vi "multifunc_scmos_frame_acquisition.vi"() -> ()   [LabVIEW 2015]
uses:
  <vilib>/Utility/miscctls.llb/LVRectTypeDef.ctl
panel:
  out "Start Trigger Mode":string
  in  "Stop Button":bool
  out "error out":errorcluster
  out "Plot Area Bounds":T1
  out "Image":u16[][](graph)
  in  "Exposure":dbl min=0.0010036691729323308 max=10.000004210526315 step=1e-08
  in  "Scan Mode":dbl min=1.0 max=2.0 step=1.0
  in  "Binning":u16(ring) items=["1x1"=1, "2x2"=2, "4x4"=4]
  out "Exposure":dbl
  out "Scan Mode":dbl
  out "S Vert Width":i32
  out "S Horiz Width":i32
  out "S Vert Offset":i32
  out "S Horiz Offset":i32
  in  "Vertical Width":i32 min=4 max=2048 step=4
  in  "Vertical Offset":i32 min=0 max=0 step=4
  in  "Horizontal Width":i32 min=4 max=2048 step=4
  in  "Horizontal Offset":i32 min=0 max=0 step=4
  in  "Frames":dbl
  out "Timeseries Save Path":path
  out "Snapshot Save Path":path
  out "Timeseries Base Filename":string
  out "Snapshot Base Filename":string
  in  "Timeseries Base Filename":string
  in  "Timeseries Save Path":path
  in  "Snapshot Base Filename":string
  in  "Save Snapshots":bool caption="Save Snapshot"
  in  "Snapshot Save Path":path
  in  "Start Trigger Mode":u32(ring)=1 items=["Internal"=1, "External Edge"=2, "External Level"=4, "Software"=32, "Fast Repetition"=64, "TDI"=128, "Trigger Start"=512, "Sync Readout"=1024]
  out "Model":string
  out "Camera ID":string
  out "Firmware":string
  out "DCAM Ver.":string
  out "Library Ver.":string
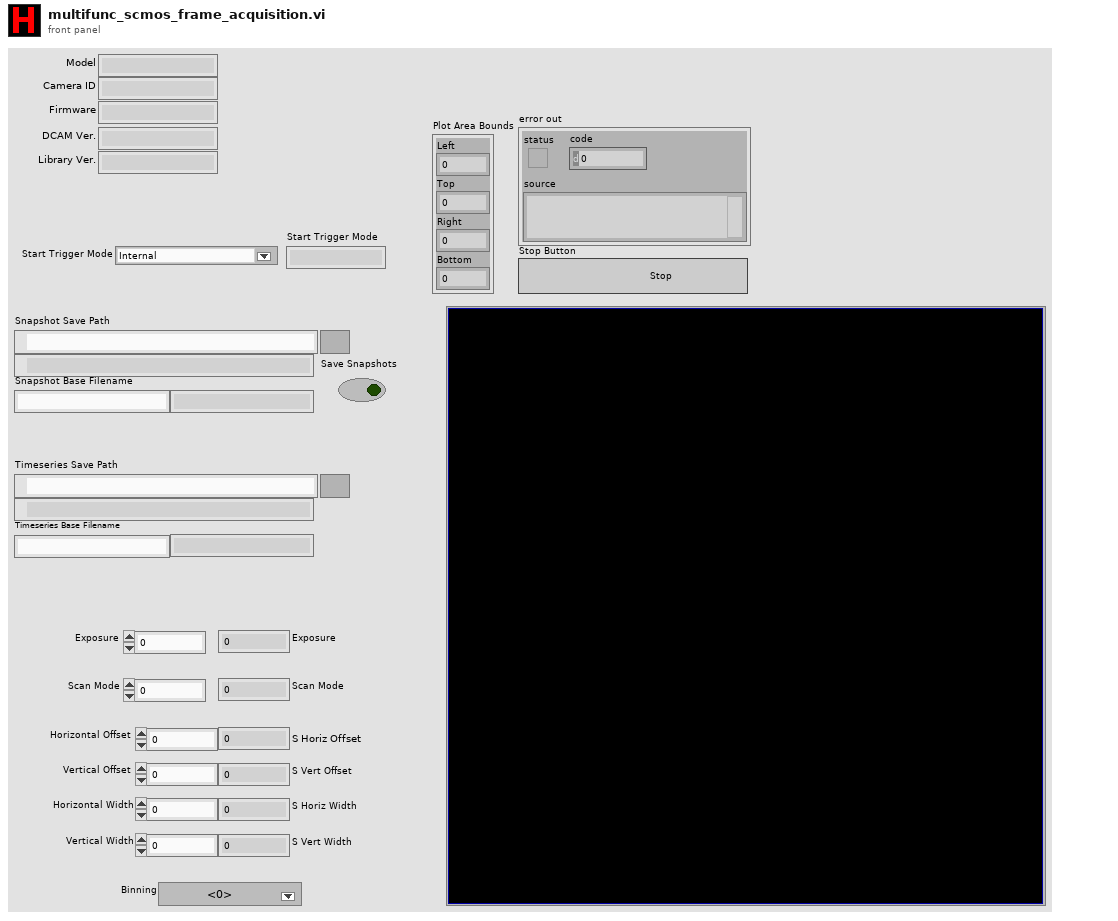
[diagram p1: front panel]
types:
  T1 = typedef "LVRectTypeDef.ctl" = cluster{"Left":i16, "Top":i16, "Right":i16, "Bottom":i16}
  T2 = cluster{"Capture Library":string, "DCAM-API":string}
  T3 = cluster{"Mode":u32, "Polarity":u16, "Times":u32, "Delay":dbl}
  T4 = cluster{"Mode":u32, "Polarity":u32, "Period":dbl, "Delay":dbl}
  T5 = cluster{"Model":string, "Camera ID":string, "Firmware":string}
  T6 = cluster{"Value":i32, "Minimum":i32, "Maximum":i32, "Increment":i32}
  T7 = cluster{"height":u32, "width":u32, "datatype":u32}
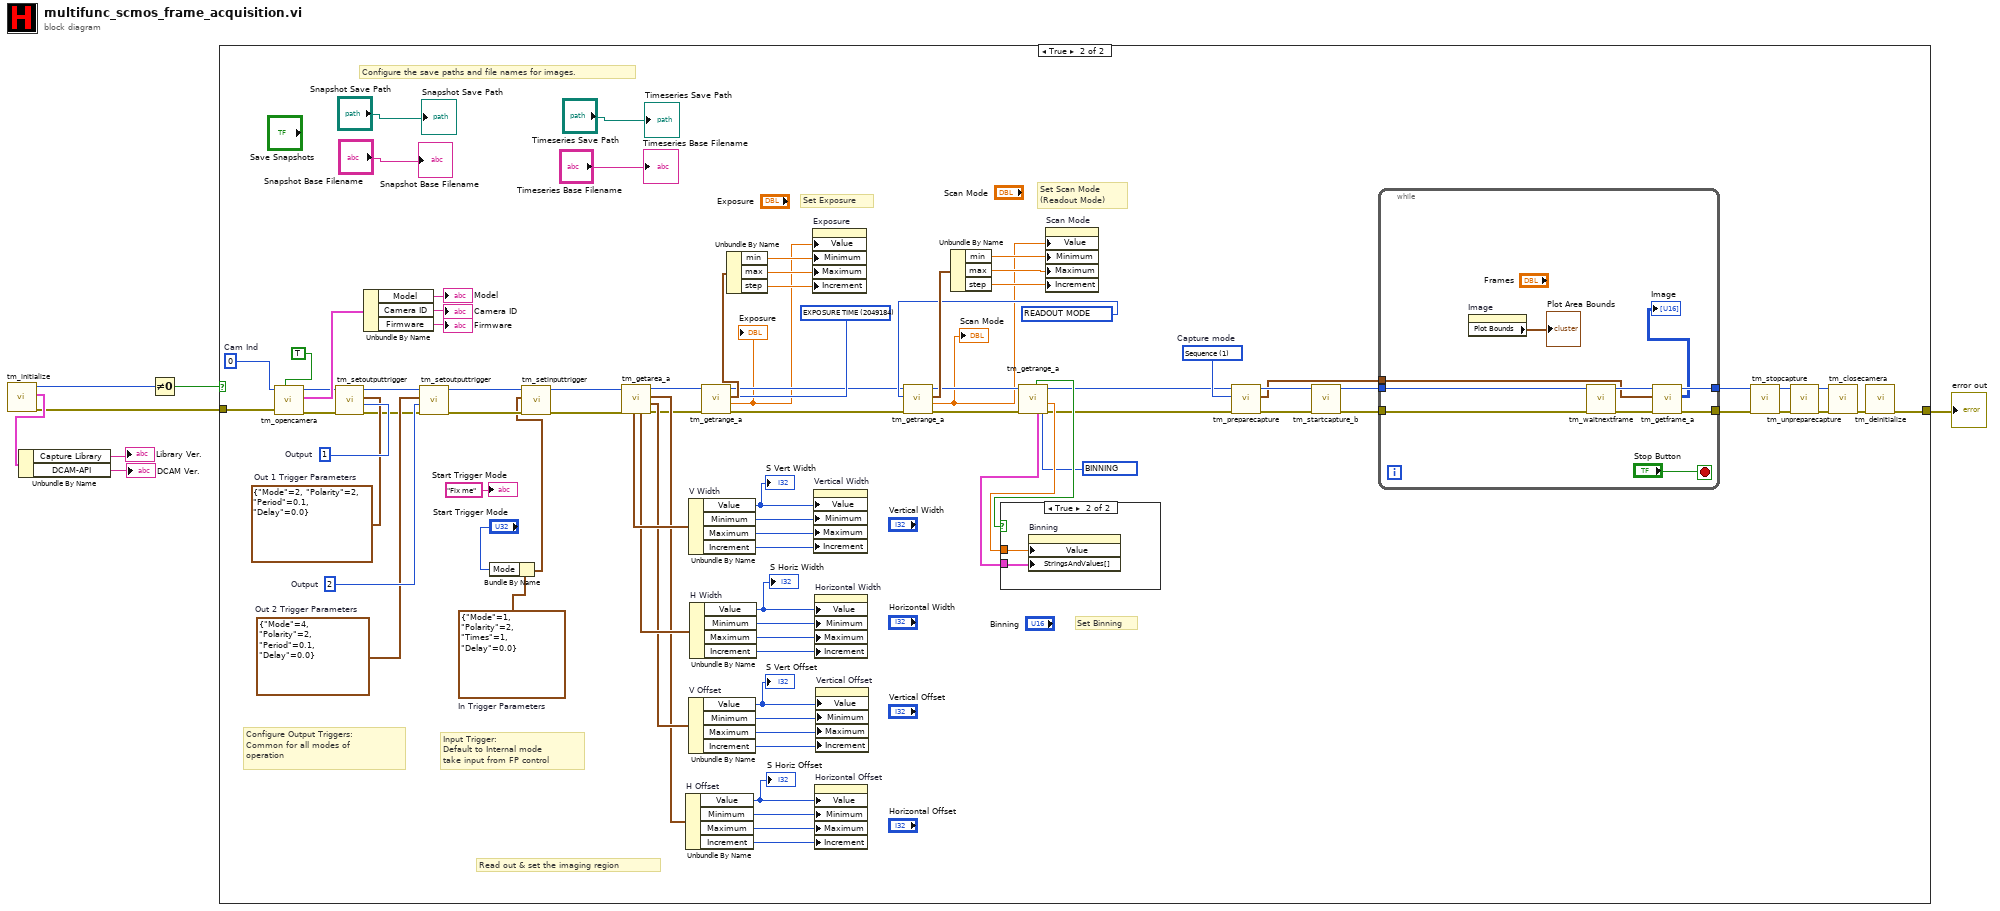
[diagram p0: block diagram]
diagram:
  n1 = call <userlib>:"tm_initialize.vi"() -> ("error out"=w3:errorcluster, "Version Info"=w4:T2, "Number Of Cameras"=w7:u32)  [unwired: 8 in, 1 out]
  n2 = Unbundle By Name(w4) -> ("Capture Library"=→"Library Ver.":string, "DCAM-API"=→"DCAM Ver.":string)
  n3 = Not Equal To 0?(x=w7) -> (x != 0?=w2:bool)
  n4 = case shown="True" w2 {
    tunnel: w3 -> [w8 w80]
    tunnel: [w8 w32] -> w1
    frame False {
    }
    frame True {
      w15 = 1 items=["Snap", "Sequence"]  # Capture mode
      w42 = u32 2049184 items=["BINNING"=4215968, "BITS PER CHANNEL"=4342976, "ACTIVE VIEW INDEX"=4343136, "CCD MODE"=4212384, "SENSOR MODE"=4212128, "READOUT MODE"=4211872, "EXPOSURE TIME"=2049184, "CONTRAST GAIN"=3163312, "CONTRAST OFFSET"=3163328, "LIGHT MODE"=2114720, "SENSITIVITY"=2114992, "WHITE BALANCE"=3163568, "PHOTON IMAGING MODE"=2115200, "HIGH DYNAMIC RANGE MODE"=3163360, "TRIGGER SOURCE"=1066144, "TRIGGER ACTIVE"=1066160, "TRIGGER MODE"=1066400, "TRIGGER POLARITY"=1066416, "TRIGGER GLOBAL EXPOSURE"=2049680, "FIRST TRIGGER BEHAVIOR"=2049696, "TRIGGER TIMES"=1066448, "OUTPUT TRIGGER POLARITY"=1852592, "OUTPUT TRIGGER DELAY"=1852624, "OUTPUT TRIGGER PERIOD"=1852640, "TEMPERATURE"=2115232, "TEMPERATURE TARGET"=2115264, "SENSOR COOLER FAN"=2115296, "MECHANICAL SHUTTER"=2115488, "BACK FOCUS POSITION"=8422304, "FRAMEBUNDLE MODE"=4346784, "FRAMEBUNDLE NUMBER"=4346800, "LINEBUNDLE HEIGHT"=4212192, "TRIGGER CONNECTOR"=1066432, "IMAGE PIXEL TYPE"=4343296, "OUTPUT TRIGGER KIND"=1852656, "READOUT DIRECTION"=4211904, "CHANNEL SYNC"=1852352] ("Parameter")
      w43 = u32 4211872 items=["BINNING"=4215968, "BITS PER CHANNEL"=4342976, "ACTIVE VIEW INDEX"=4343136, "CCD MODE"=4212384, "SENSOR MODE"=4212128, "READOUT MODE"=4211872, "EXPOSURE TIME"=2049184, "CONTRAST GAIN"=3163312, "CONTRAST OFFSET"=3163328, "LIGHT MODE"=2114720, "SENSITIVITY"=2114992, "WHITE BALANCE"=3163568, "PHOTON IMAGING MODE"=2115200, "HIGH DYNAMIC RANGE MODE"=3163360, "TRIGGER SOURCE"=1066144, "TRIGGER ACTIVE"=1066160, "TRIGGER MODE"=1066400, "TRIGGER POLARITY"=1066416, "TRIGGER GLOBAL EXPOSURE"=2049680, "FIRST TRIGGER BEHAVIOR"=2049696, "TRIGGER TIMES"=1066448, "OUTPUT TRIGGER POLARITY"=1852592, "OUTPUT TRIGGER DELAY"=1852624, "OUTPUT TRIGGER PERIOD"=1852640, "TEMPERATURE"=2115232, "TEMPERATURE TARGET"=2115264, "SENSOR COOLER FAN"=2115296, "MECHANICAL SHUTTER"=2115488, "BACK FOCUS POSITION"=8422304, "FRAMEBUNDLE MODE"=4346784, "FRAMEBUNDLE NUMBER"=4346800, "LINEBUNDLE HEIGHT"=4212192, "TRIGGER CONNECTOR"=1066432, "IMAGE PIXEL TYPE"=4343296, "OUTPUT TRIGGER KIND"=1852656, "READOUT DIRECTION"=4211904, "CHANNEL SYNC"=1852352] ("Parameter")
      w44 = u32 4215968 items=["BINNING"=4215968, "BITS PER CHANNEL"=4342976, "ACTIVE VIEW INDEX"=4343136, "CCD MODE"=4212384, "SENSOR MODE"=4212128, "READOUT MODE"=4211872, "EXPOSURE TIME"=2049184, "CONTRAST GAIN"=3163312, "CONTRAST OFFSET"=3163328, "LIGHT MODE"=2114720, "SENSITIVITY"=2114992, "WHITE BALANCE"=3163568, "PHOTON IMAGING MODE"=2115200, "HIGH DYNAMIC RANGE MODE"=3163360, "TRIGGER SOURCE"=1066144, "TRIGGER ACTIVE"=1066160, "TRIGGER MODE"=1066400, "TRIGGER POLARITY"=1066416, "TRIGGER GLOBAL EXPOSURE"=2049680, "FIRST TRIGGER BEHAVIOR"=2049696, "TRIGGER TIMES"=1066448, "OUTPUT TRIGGER POLARITY"=1852592, "OUTPUT TRIGGER DELAY"=1852624, "OUTPUT TRIGGER PERIOD"=1852640, "TEMPERATURE"=2115232, "TEMPERATURE TARGET"=2115264, "SENSOR COOLER FAN"=2115296, "MECHANICAL SHUTTER"=2115488, "BACK FOCUS POSITION"=8422304, "FRAMEBUNDLE MODE"=4346784, "FRAMEBUNDLE NUMBER"=4346800, "LINEBUNDLE HEIGHT"=4212192, "TRIGGER CONNECTOR"=1066432, "IMAGE PIXEL TYPE"=4343296, "OUTPUT TRIGGER KIND"=1852656, "READOUT DIRECTION"=4211904, "CHANNEL SYNC"=1852352] ("Parameter")
      w75 = T3 {"Mode"=1, "Polarity"=2, "Times"=1, "Delay"=0.0}  # In Trigger Parameters
      w81 = T4 {"Mode"=4, "Polarity"=2, "Period"=0.1, "Delay"=0.0}  # Out 2 Trigger Parameters
      w82 = T4 {"Mode"=2, "Polarity"=2, "Period"=0.1, "Delay"=0.0}  # Out 1 Trigger Parameters
      w84 = 2  # Output
      w86 = 1  # Output
      w92 = 0  # Cam Ind
      # "Configure the save paths and file names for images."
      # "Set Binning"
      # "Set Scan Mode \n(Readout Mode)"
      # "Set Exposure"
      # "Read out & set the imaging region"
      # "Input Trigger:\nDefault to Internal mode\ntake input from FP control"
      # "Configure Output Triggers: \nCommon for all modes of operation"
      n5 = call <userlib>:"tm_opencamera.vi"("Force Open"=TRUE, "error in (no error)"=w80, "Camera Index"=w92) -> ("error out"=w79:errorcluster, "Camera Details"=w91:T5, "Handle out"=w87:u32)  [unwired: 6 in]
      n6 = call <userlib>:"tm_setoutputtrigger.vi"("error in (no error)"=w79, "Index"=w86, "Parameters"=w82) -> ("error out"=w78:errorcluster, "Handle out"=w85:u32)  [unwired: 7 in]
      n7 = Unbundle By Name(w91) -> ("Model"=→"Model":string, "Camera ID"=→"Camera ID":string, "Firmware"=→"Firmware":string)
      n8 = call <userlib>:"tm_setoutputtrigger.vi"("error in (no error)"=w78, "Index"=w84, "Parameters"=w81, "Handle in"=w85) -> ("error out"=w77:errorcluster)  [unwired: 6 in, 1 out]
      n9 = Bundle By Name(cluster=w75, "Mode"="Start Trigger Mode") -> (w76:T3)
      n10 = call <userlib>:"tm_setinputtrigger.vi"("error in (no error)"=w77, "Parameters"=w76, "Handle in"=w87) -> ("error out"=w72:errorcluster, "Handle out"=w73:u32)  [unwired: 7 in]
      n11 = call <userlib>:"tm_getarea_a.vi"("error in (no error)"=w72, "Handle in"=w73) -> ("error out"=w41:errorcluster, "V Offset"=w69:T6, "H Offset"=w68:T6, "Handle out"=w40:u32, "H Width"=w70:T6, "V Width"=w71:T6)  [unwired: 4 in]
      n12 = Unbundle By Name "H Offset"(w68) -> ("Value"=w55:i32, "Minimum"=w54:i32, "Maximum"=w53:i32, "Increment"=w52:i32)
      "S Horiz Offset" <- w55
      n13 = Unbundle By Name "V Width"(w71) -> ("Value"=w67:i32, "Minimum"=w66:i32, "Maximum"=w65:i32, "Increment"=w64:i32)
      "S Vert Width" <- w67
      n14 = Unbundle By Name "V Offset"(w69) -> ("Value"=w59:i32, "Minimum"=w58:i32, "Maximum"=w57:i32, "Increment"=w56:i32)
      "S Vert Offset" <- w59
      n15 = Unbundle By Name "H Width"(w70) -> ("Value"=w63:i32, "Minimum"=w62:i32, "Maximum"=w61:i32, "Increment"=w60:i32)
      "S Horiz Width" <- w63
      n16 = call <userlib>:"tm_getrange_a.vi"("error in (no error)"=w41, "Parameter"=w42, "Handle in"=w40) -> ("error out"=w50:errorcluster, "default"=w26:dbl, "Range"=w51:cluster{"min":dbl, "max":dbl, "step":dbl}, "Handle out"=w39:u32)  [unwired: 2 in, 3 out]
      "Exposure" <- w26
      n17 = Unbundle By Name(w51) -> ("min"=w27:dbl, "max"=w28:dbl, "step"=w29:dbl)
      n18 = property on="Exposure" class="DigNum (strict)"("Value"=w26, "Minimum"=w27, "Maximum"=w28, "Increment"=w29) -> ()  [unwired: 2 in, 2 out]
      n19 = property on="Vertical Width" class="DigNum (strict)"("Value"=w67, "Minimum"=w66, "Maximum"=w65, "Increment"=w64) -> ()  [unwired: 2 in, 2 out]
      n20 = property on="Horizontal Width" class="DigNum (strict)"("Value"=w63, "Minimum"=w62, "Maximum"=w61, "Increment"=w60) -> ()  [unwired: 2 in, 2 out]
      n21 = property on="Horizontal Offset" class="DigNum (strict)"("Value"=w55, "Minimum"=w54, "Maximum"=w53, "Increment"=w52) -> ()  [unwired: 2 in, 2 out]
      n22 = property on="Vertical Offset" class="DigNum (strict)"("Value"=w59, "Minimum"=w58, "Maximum"=w57, "Increment"=w56) -> ()  [unwired: 2 in, 2 out]
      n23 = call <userlib>:"tm_getrange_a.vi"("error in (no error)"=w50, "Parameter"=w43, "Handle in"=w39) -> ("error out"=w48:errorcluster, "default"=w22:dbl, "Range"=w49:cluster{"min":dbl, "max":dbl, "step":dbl}, "Handle out"=w38:u32)  [unwired: 2 in, 3 out]
      "Scan Mode" <- w22
      n24 = Unbundle By Name(w49) -> ("min"=w23:dbl, "max"=w24:dbl, "step"=w25:dbl)
      n25 = call <userlib>:"tm_getrange_a.vi"("error in (no error)"=w48, "Parameter"=w44, "Handle in"=w38) -> ("error out"=w12:errorcluster, "default"=w46:dbl, "Handle out"=w13:u32, "Value Names"=w45:cluster{"Name":string, "Value":dbl}[], "Writable"=w47:bool)  [unwired: 2 in, 2 out]
      n26 = case shown="True" w47 {
        tunnel: w45 -> [_ w103]
        tunnel: w46 -> [_ w104]
        frame False {
        }
        frame True {
          n27 = property on="Binning" class="Ring (strict)"("Value"=w104, "StringsAndValues[]"=w103) -> ()  [unwired: 2 in, 2 out]
        }
      }
      n28 = property on="Scan Mode" class="DigNum (strict)"("Value"=w22, "Minimum"=w23, "Maximum"=w24, "Increment"=w25) -> ()  [unwired: 2 in, 2 out]
      n29 = call <userlib>:"tm_preparecapture.vi"("error in (no error)"=w12, "Capture mode"=w15, "Handle in"=w13) -> ("error out"=w16:errorcluster, "Buffer Info"=w14:T7, "Handle out"=w17:u32)  [unwired: 5 in, 1 out]
      n30 = call <userlib>:"tm_startcapture_b.vi"("error in (no error)"=w16, "Handle in"=w17) -> ("error out"=w11:errorcluster, "Handle out"=w10:u32)  [unwired: 8 in]
      n31 = while {
        tunnel: w10 -> [w95]
        tunnel: [w99] -> w30
        tunnel: w11 -> [w94]
        tunnel: [w100] -> w31
        tunnel: w14 -> [w93]
        stop <- "Stop Button" stop-if-true
        n32 = property on="Image" class="IntGraph (strict)"() -> ("Plot Bounds"=→"Plot Area Bounds":T1)  [unwired: 2 in, 2 out]
        n33 = call <userlib>:"tm_waitnextframe.vi"("error in (no error)"=w94, "Handle in"=w95) -> ("error out"=w101:errorcluster, "Handle out"=w102:u32)  [unwired: 6 in, 2 out]
        n34 = call <userlib>:"tm_getframe_a.vi"("error in (no error)"=w101, "Buffer Info"=w93, "Handle in"=w102) -> ("error out"=w100:errorcluster, "Data 16"=→"Image":u16[][], "Handle out"=w99:u32)  [unwired: 4 in, 2 out]
      }
      n35 = call <userlib>:"tm_stopcapture.vi"("error in (no error)"=w31, "Handle in"=w30) -> ("error out"=w36:errorcluster, "Handle out"=w35:u32)  [unwired: 8 in]
      n36 = call <userlib>:"tm_unpreparecapture.vi"("error in (no error)"=w36, "Handle in"=w35) -> ("error out"=w37:errorcluster, "Handle out"=w34:u32)  [unwired: 8 in]
      n37 = call <userlib>:"tm_closecamera.vi"("error in (no error)"=w37, "Handle in"=w34) -> ("error out"=w33:errorcluster)  [unwired: 9 in]
      n38 = call <userlib>:"tm_deinitialize.vi"("error in (no error)"=w33) -> ("error out"=w32:errorcluster)  [unwired: 10 in]
      "Timeseries Base Filename" <- "Timeseries Base Filename"
      "Timeseries Save Path" <- "Timeseries Save Path"
      "Snapshot Base Filename" <- "Snapshot Base Filename"
      "Snapshot Save Path" <- "Snapshot Save Path"
      "Start Trigger Mode" <- "Fix me"
    }
  }
  "error out" <- w1
